vi "Extended Rosenbrock Function.vi"(3 "output control":T1, 4 "data":variant, 5 "X":dbl[](array[numeric])) -> (0 "error out":errorcluster, 1 "gradient":dbl[](array[numeric]), 2 "f(X)":dbl)   [LabVIEW 2016]
doc: "Use this template VI as a starting point to create an objective function you want to pass to the Unconstrained Optimization VI."
uses:
  <vilib>/Utility/error.llb/Error Cluster From Error Code.vi
  <vilib>/ErrorRing/Error Ring.xnode
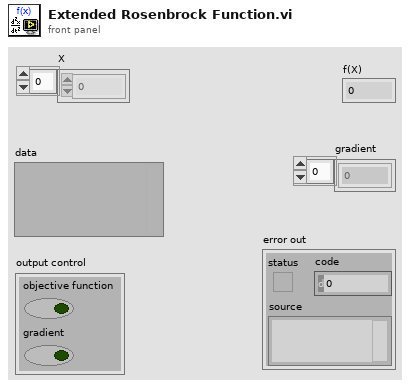
[diagram p1: front panel]
types:
  T1 = cluster{"objective function":bool, "gradient":bool}
  T2 = cluster{"c":dbl, "Intensity Graph":refnum<vi>, "animate?":bool}
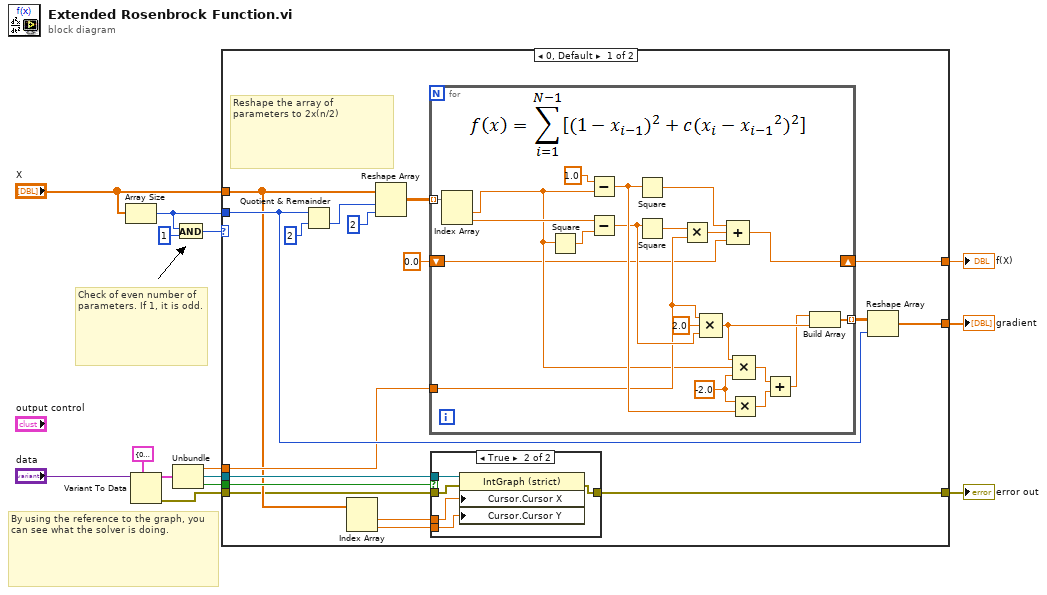
[diagram p0: block diagram]
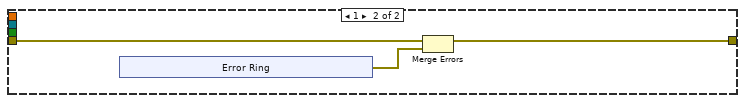
[diagram p3: hidden frame]
diagram:
  # "By using the reference to the graph, you can see what the solver is doing."
  # "Check of even number of parameters. If 1, it is odd."
  n1 = Array Size(array="X") -> (size(s)=w10:i32)
  n2 = Variant To Data(type=T2 {"c"=0.0, "Intensity Graph"=refnum, "animate?"=FALSE} ("output cluster"), Variant="data") -> (data=w6:T2, error out=w1:errorcluster)  [unwired: 1 in]
  n3 = Unbundle(w6) -> ("c"=w4:dbl, "Intensity Graph"=w3:refnum<vi>, "animate?"=w2:bool)
  n4 = And(x=w10, y=1) -> (x .and. y?=w13:i32)
  n5 = case shown="0, Default" w13 {
    tunnel: [w15 w59] -> w12
    tunnel: "X" -> [w19 _]
    tunnel: w10 -> [w24 _]
    tunnel: [w26 _] -> w9
    tunnel: [w23 _] -> w8
    tunnel: w4 -> [w22 _]
    tunnel: w3 -> [w21 _]
    tunnel: w2 -> [w20 _]
    tunnel: w1 -> [w16 w60]
    frame 0, Default {
      # "Reshape the array of parameters to 2x(n/2)"
      n6 = Quotient & Remainder(x=w24, y=2) -> (floor(x/y)=w30:i32)  [unwired: 1 out]
      n7 = Index Array(array=w19) -> (element #1=w18:dbl, element #2=w17:dbl)  [unwired: 2 in]
      n8 = Reshape Array(w19, w30, 2 ("dimension size")) -> (w28:dbl[][])
      n9 = for {
        tunnel: w28 -> [w57] mode=indexing
        shift-right: [w51] -> w26
        shift-left: 0.0 -> [w38]
        tunnel: [w44] -> w25 mode=indexing
        tunnel: w22 -> [w41]
        w40 = -2.0 ("value")
        n10 = Index Array(array=w57) -> (element #1=w39:dbl, element #2=w43:dbl)  [unwired: 2 in]
        n11 = Square(x=w39) -> (x^2=w56:dbl)
        n12 = Subtract(x=1.0, y=w39) -> (x-y=w49:dbl)
        n13 = Subtract(x=w43, y=w56) -> (x-y=w42:dbl)
        n14 = Square(x=w49) -> (x^2=w52:dbl)
        n15 = Square(x=w42) -> (x^2=w55:dbl)
        n16 = Multiply(x=w55, y=w41) -> (x*y=w54:dbl)
        n17 = Compound Arithmetic op=MULTIPLY(w41, 2.0, w42) -> (w48:dbl)
        n18 = Compound Arithmetic op=ADD(w52, w54, w38) -> (w51:dbl)
        n19 = Multiply(x=w40, y=w49) -> (x*y=w46:dbl)
        n20 = Compound Arithmetic op=MULTIPLY(w48, w39, w40) -> (w47:dbl)
        n21 = Add(x=w47, y=w46) -> (x+y=w45:dbl)
        n22 = Build Array(w45, w48) -> (w44:dbl[])
      }
      n23 = case shown="True" w20 {
        tunnel: w21 -> [_ w37]
        tunnel: w18 -> [_ w36]
        tunnel: w17 -> [_ w35]
        tunnel: w16 -> [w32 w34]
        tunnel: [w32 w33] -> w15
        frame False {
        }
        frame True {
          n24 = property on="Property Node" class="IntGraph (strict)"(reference=w37, error in=w34, "Cursor.Cursor X"=w36, "Cursor.Cursor Y"=w35) -> (error out=w33:errorcluster)  [unwired: 1 out]
        }
      }
      n25 = Reshape Array(w25, w24) -> (w23:dbl[])
    }
    frame 1 {
      n26 = xnode "Error Ring"() -> ("error out"=w58:errorcluster)
      n27 = Merge Errors(w60, w58) -> (w59:errorcluster)
    }
  }
  "error out" <- w12
  "f(X)" <- w9
  "gradient" <- w8
